vi "preScanHoldtime.vi"(8 "error in (no error)":errorcluster, 11 "ChirpWave in":refnum<class "ChirpWave.lvclass">) -> (0 "error out":errorcluster, 2 "PrescanHold?":bool=TRUE, 3 "ChirpWave out":refnum<class "ChirpWave.lvclass">)   [LabVIEW 2015, in "ChirpWave.lvclass"]
uses:
  ChirpWave.lvclass
  ChirpWave.lvclass/ChirpWave.ctl
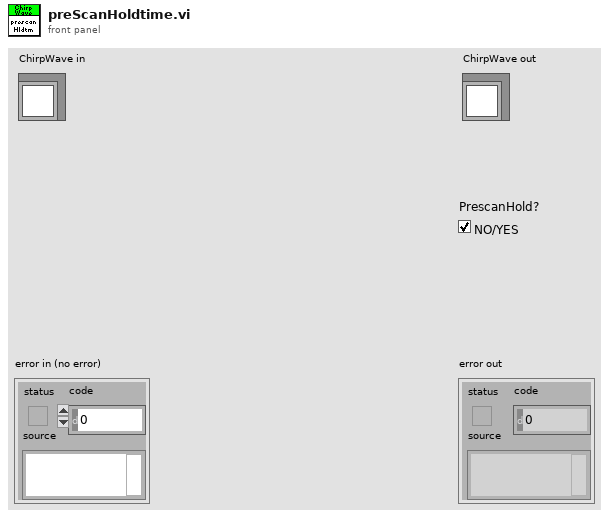
[diagram p1: front panel]
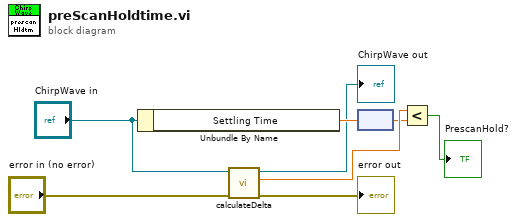
[diagram p0: block diagram]
diagram:
  n1 = Unbundle By Name("ChirpWave in") -> ("Settling Time"=w6:dbl[unit])
  n2 = call "calculateDelta.vi"("error in (no error)"="error in (no error)", "ChirpWave in"="ChirpWave in") -> ("error out"=→"error out":errorcluster, "Delta Timestamp"=w8:dbl, "ChirpWave out"=→"ChirpWave out":refnum<class "ChirpWave.lvclass">)  [unwired: 7 in]
  n3 = node(w6) -> (w5:dbl)
  n4 = Less?(x=w8, y=w5) -> (x < y?=→"PrescanHold?":bool)
